vi "Disable Source Trigger.vi"(8 "error in (no error)":errorcluster, 11 "Ganged Session in":T1) -> (0 "error out":errorcluster, 3 "Ganged Session out":T1)   [LabVIEW 2021]
uses:
  ctl/NIDCPower_channel_ganging - ctl - ganged session.ctl
  ctl/NIDCPower_channel_ganging - ctl - ganged config.ctl
  ctl/NIDCPower_channel_ganging - ctl - channel mode.ctl
  <instrlib>/niDCPower/nidcpower.llb/niDCPower Disable Source Trigger With Channels.vi
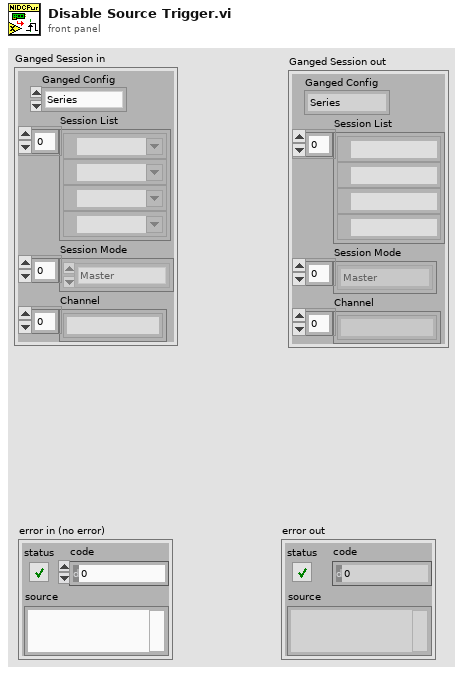
[diagram p1: front panel]
types:
  T1 = typedef "NIDCPower_channel_ganging - ctl - ganged session.ctl" = cluster{"Ganged Config":T2, "Session List":refnum<k15>[], "Session Mode":T3[], "Channel":string[]}
  T2 = typedef "NIDCPower_channel_ganging - ctl - ganged config.ctl" = enum32{"Series", "Parallel", "Manual"}
  T3 = typedef "NIDCPower_channel_ganging - ctl - channel mode.ctl" = enum32{"Master", "Slave", "Slave - Inverted"}
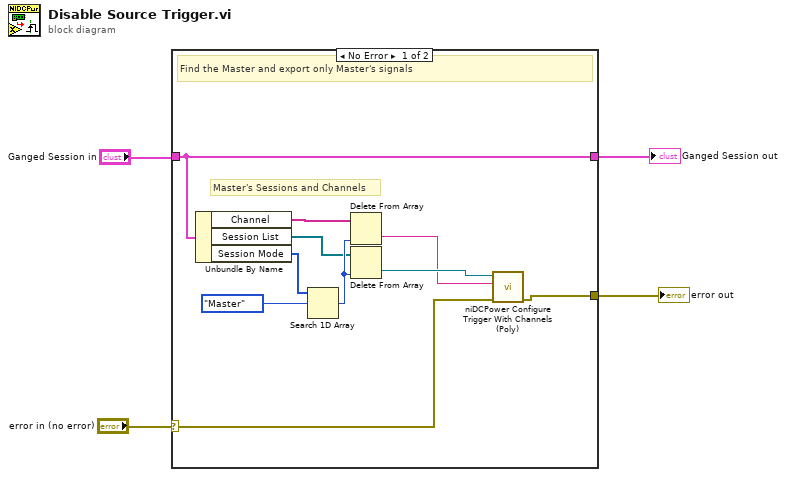
[diagram p0: block diagram]
diagram:
  n1 = case shown="No Error" "error in (no error)" {
    selector: "error in (no error)" -> [w6 w16]
    tunnel: [w5 w16] -> w4
    tunnel: "Ganged Session in" -> [w13 w15]
    tunnel: [w13 w15] -> w2
    frame No Error {
      # "Master's Sessions and Channels"
      # "Find the Master and export only Master's signals"
      n2 = Unbundle By Name(w13) -> ("Channel"=w11:string[], "Session List"=w10:refnum<k15>[], "Session Mode"=w9:T3[])
      n3 = Search 1D Array(1D array=w9, element=NIDCPower_channel_ganging_-_ctl_-_channel_mode."Master" ("Channel Mode")) -> (index of element=w12:i32)  [unwired: 1 in]
      n4 = Delete From Array(array=w11, index=w12) -> (deleted portion=w7:string)  [unwired: 1 in, 1 out]
      n5 = Delete From Array(array=w10, index=w12) -> (deleted portion=w8:refnum<k15>)  [unwired: 1 in, 1 out]
      n6 = call-poly <instrlib>:"niDCPower Configure Trigger With Channels (Poly).vi"("error in (no error)"=w6, "channel name"=w7, "instrument handle"=w8) -> ("error out"=w5:errorcluster)  [unwired: 7 in, 1 out]
    }
    frame Error {
    }
  }
  "error out" <- w4
  "Ganged Session out" <- w2
